vi "Resolve (String).vi"(8 "error in (no error)":errorcluster, 10 "Element":refnum<class "Config Element.lvclass">, 11 "Sequence Constants in":refnum<class "Sequence Constants.lvclass">) -> (0 "error out":errorcluster, 2 "String Value":string, 3 "Sequence Constants out":refnum<class "Sequence Constants.lvclass">)   [LabVIEW 2020, in "VolatusSeqConfig.lvlib" / "Sequence Constants.lvclass"]
uses:
  Sequence Constants.lvclass
  lv-cdm/CDM-Config/Config Element/Config Element.lvclass
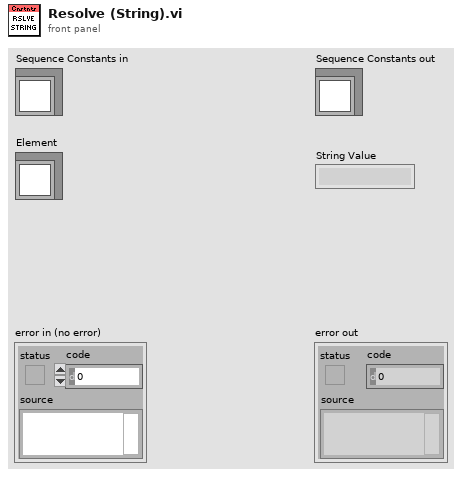
[diagram p1: front panel]
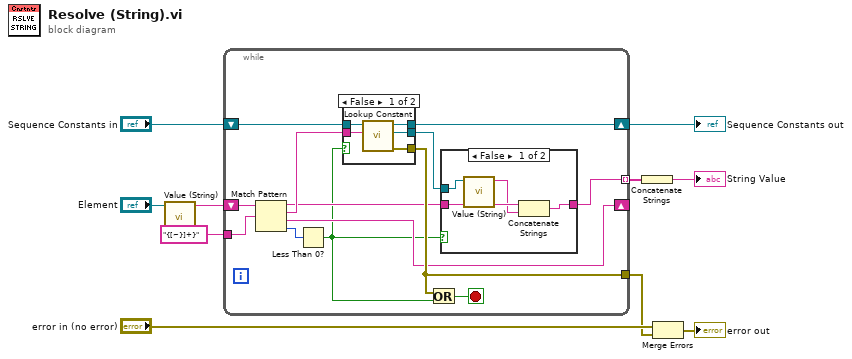
[diagram p0: block diagram]
diagram:
  n1 = call "Value (String).vi"("Config Element in"="Element") -> ("String Value"=w7:string)  [unwired: 9 in, 1 out]
  n2 = while {
    shift-right: [w14] -> _
    shift-left: w7 -> [w22]
    tunnel: "{[~}]+}" ("regular expression") -> [w21]
    tunnel: [w23] -> w4
    shift-right: [w16] -> w5
    shift-left: "Sequence Constants in" -> [w12]
    tunnel: [w13] -> w2 mode=indexing
    stop <- w17 stop-if-true
    n3 = Match Pattern(string=w22, regular expression=w21) -> (before substring=w15:string, match substring=w20:string, after substring=w14:string, offset past match=w19:i32)  [unwired: 1 in]
    n4 = Less Than 0?(x=w19) -> (x < 0?=w11:bool)
    n5 = case shown="False" w11 {
      tunnel: w20 -> [w28 _]
      tunnel: [w27 _] -> w18
      tunnel: [w26 w29] -> w16
      tunnel: w12 -> [w25 w29]
      tunnel: [w24 _] -> w23
      frame False {
        n6 = call "Lookup Constant.vi"("Constant Name"=w28, "Sequence Constants in"=w25) -> ("error out"=w24:errorcluster, "Element"=w27:refnum<class "Config Element.lvclass">, "Sequence Constants out"=w26:refnum<class "Sequence Constants.lvclass">)  [unwired: 7 in]
      }
      frame True {
      }
    }
    n7 = Or(x=w23, y=w11) -> (x .or. y?=w17:bool)
    n8 = case shown="False" w11 {
      tunnel: w15 -> [w32 w34]
      tunnel: w18 -> [w33 _]
      tunnel: [w30 w34] -> w13
      frame False {
        n9 = call "Value (String).vi"("Config Element in"=w33) -> ("String Value"=w31:string)  [unwired: 9 in, 1 out]
        n10 = Concatenate Strings(w32, w31) -> (w30:string)
      }
      frame True {
      }
    }
  }
  "Sequence Constants out" <- w5
  n11 = Concatenate Strings(w2) -> (→"String Value":string)
  n12 = Merge Errors("error in (no error)", w4) -> (→"error out":errorcluster)
